vi "obstacle.vi"(3 "width":dbl) -> (0 "down":dbl, 1 "up":dbl)   [LabVIEW 2014]
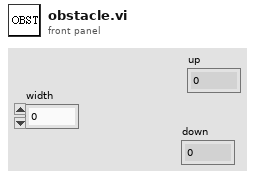
[diagram p1: front panel]
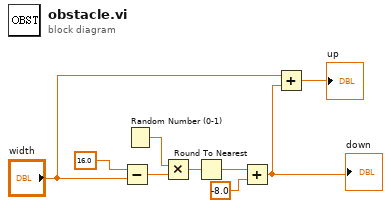
[diagram p0: block diagram]
diagram:
  n1 = Subtract(x=16.0, y="width") -> (x-y=w8:dbl)
  n2 = Random Number (0-1)() -> (number: 0 to 1=w7:dbl)
  n3 = Multiply(x=w7, y=w8) -> (x*y=w6:dbl)
  n4 = Round To Nearest(number=w6) -> (nearest integer value=w5:dbl)
  n5 = Add(x=w5, y=-8.0) -> (x+y=w2:dbl)
  "down" <- w2
  n6 = Add(x="width", y=w2) -> (x+y=→"up":dbl)
